vi "模拟时钟.vi"() -> ()   [LabVIEW 2016]
panel:
  out "时钟绘图":picture
  out "时间字符串":string
types:
  T1 = cluster{"Width":u16, "Style":enum32{"Solid", "Dash", "Dot", "DashDot", "DashDotDot"}}
  T2 = typedef "LVBoundsTypeDef.ctl" = cluster{"Width":u32, "Height":u32}
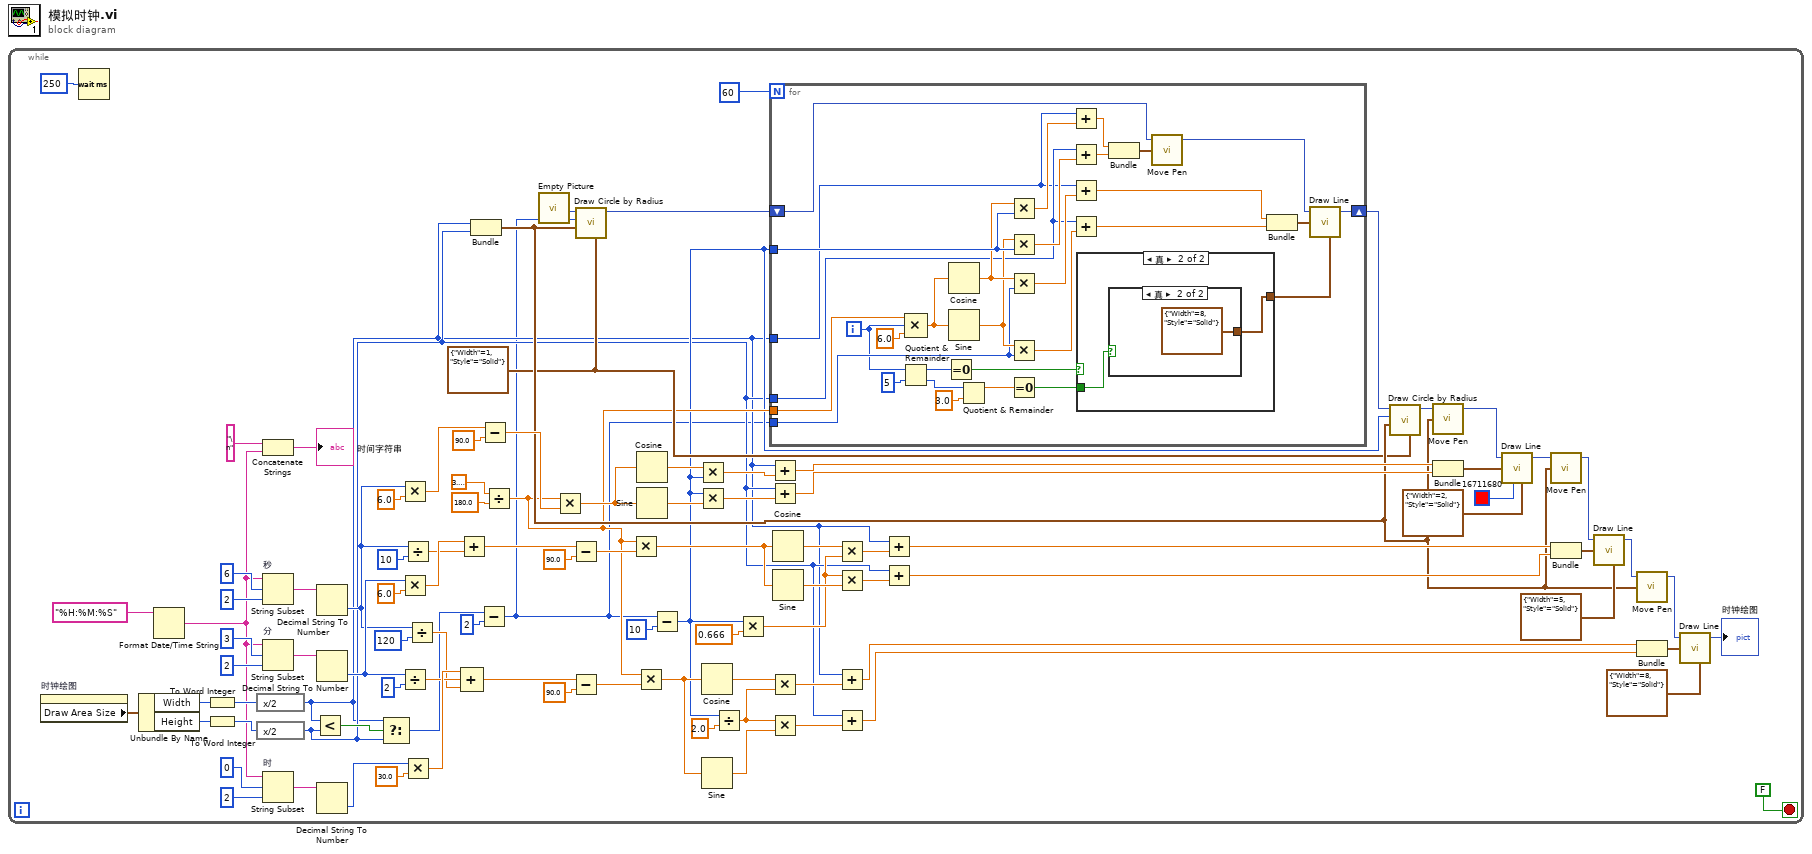
[diagram p0: block diagram]
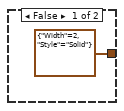
[diagram p2: hidden frame]
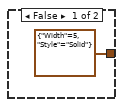
[diagram p3: hidden frame]
diagram:
  n1 = while {
    stop <- FALSE stop-if-true
    w14 = T1 {"Width"=1, "Style"=enum."Solid"} ("pen")
    n2 = property on="时钟绘图" class="Pict"() -> ("Draw Area Size"=w97:T2)  [unwired: 2 in, 2 out]
    n3 = Wait (ms)(milliseconds to wait=u32 250 ("等待时间（毫秒）")) -> ()  [unwired: 1 out]
    n4 = Unbundle By Name(w97) -> ("Width"=w93:u32, "Height"=w92:u32)
    n5 = Format Date/Time String(time format string (%c)="%H:%M:%S" ("时间格式字符串(%c)")) -> (date/time string=w3:string)  [unwired: 2 in]
    n6 = To Word Integer(number=w93) -> (16bit integer=w90:i16)
    n7 = To Word Integer(number=w92) -> (16bit integer=w89:i16)
    n8 = expression code="x/2"(w90) -> (w7:i16)
    n9 = expression code="x/2"(w89) -> (w8:i16)
    n10 = Concatenate Strings("\n" ("字符串"), w3) -> (→"时间字符串":string)
    n11 = String Subset "秒"(string=w3, offset (0)=6 ("偏移量(0)"), length (rest)=2 ("长度（剩余）")) -> (substring=w78:string)
    n12 = String Subset "分"(string=w3, offset (0)=3 ("偏移量(0)"), length (rest)=2 ("长度（剩余）")) -> (substring=w81:string)
    n13 = String Subset "时"(string=w3, offset (0)=0 ("偏移量(0)"), length (rest)=2 ("长度（剩余）")) -> (substring=w73:string)
    n14 = Less?(x=w7, y=w8) -> (x < y?=w94:bool)
    n15 = Decimal String To Number(string=w78) -> (number=w31:i32)  [unwired: 2 in, 1 out]
    n16 = Decimal String To Number(string=w81) -> (number=w35:i32)  [unwired: 2 in, 1 out]
    n17 = Decimal String To Number(string=w73) -> (number=w36:i32)  [unwired: 2 in, 1 out]
    n18 = Select(t=w7, s=w94, f=w8) -> (s? t:f=w13:i16)
    n19 = Multiply(x=w31, y=6.0) -> (x*y=w68:dbl)
    n20 = Multiply(x=w35, y=6.0) -> (x*y=w61:dbl)
    n21 = Divide(x=w35, y=2) -> (x/y=w33:dbl)
    n22 = Divide(x=w31, y=10) -> (x/y=w60:dbl)
    n23 = Multiply(x=w36, y=30.0) -> (x*y=w37:dbl)
    n24 = Divide(x=w31, y=120) -> (x/y=w32:dbl)
    n25 = Add(x=w61, y=w60) -> (x+y=w62:dbl)
    n26 = Compound Arithmetic op=ADD(w37, w33, w32) -> (w39:dbl)
    n27 = Bundle(w7, w8) -> (w15:cluster{i16, i16})  [unwired: 1 in]
    n28 = Subtract(x=w13, y=i16 2) -> (x-y=w6:i16)
    n29 = Subtract(x=w68, y=90.0) -> (x-y=w71:dbl)
    n30 = Divide(x=3.141592653589793, y=180.0) -> (x/y=w10:dbl)
    n31 = call "Empty Picture"() -> ("empty picture"=w16:picture)
    n32 = Multiply(x=w10, y=w71) -> (x*y=w82:dbl)
    n33 = Subtract(x=w62, y=90.0) -> (x-y=w65:dbl)
    n34 = Subtract(x=w39, y=90.0) -> (x-y=w42:dbl)
    n35 = call <vilib>:"Draw Circle by Radius.vi"("pen"=w14, "pixel center"=w15, "radius"=w6, "picture"=w16) -> ("new picture"=w5:picture)  [unwired: 7 in]
    n36 = Multiply(x=w10, y=w65) -> (x*y=w50:dbl)
    n37 = Multiply(x=w10, y=w42) -> (x*y=w49:dbl)
    n38 = Cosine(x=w82) -> (cos(x)=w86:dbl)
    n39 = Sine(x=w82) -> (sin(x)=w88:dbl)
    n40 = Subtract(x=w6, y=i16 10) -> (x-y=w9:i16)
    n41 = Multiply(x=w86, y=w9) -> (x*y=w85:dbl)
    n42 = Multiply(x=w9, y=w88) -> (x*y=w87:dbl)
    n43 = Cosine(x=w49) -> (cos(x)=w44:dbl)
    n44 = Sine(x=w49) -> (sin(x)=w46:dbl)
    n45 = Divide(x=w9, y=2.0) -> (x/y=w22:dbl)
    n46 = Multiply(x=w9, y=0.666) -> (x*y=w20:dbl)
    n47 = for {
      N: 60 -> [_]
      tunnel: w10 -> [w130]
      tunnel: w9 -> [w127]
      tunnel: w8 -> [w112]
      tunnel: w7 -> [w111]
      tunnel: w6 -> [w120]
      shift-right: [w109] -> w4
      shift-left: w5 -> [w110]
      i -> [w105]
      n48 = Quotient & Remainder(x=w105, y=5) -> (x-y*floor(x/y)=w107:i32, floor(x/y)=w102:i32)
      n49 = Compound Arithmetic op=MULTIPLY(w130, w105, 6.0 ("y")) -> (w128:dbl)
      n50 = Equal To 0?(x=w107) -> (x = 0?=w106:bool)
      n51 = Cosine(x=w128) -> (cos(x)=w122:dbl)
      n52 = Sine(x=w128) -> (sin(x)=w121:dbl)
      n53 = Quotient & Remainder(x=w102, y=3.0) -> (x-y*floor(x/y)=w101:dbl)  [unwired: 1 out]
      n54 = Multiply(x=w122, y=w127) -> (x*y=w123:dbl)
      n55 = Multiply(x=w121, y=w127) -> (x*y=w126:dbl)
      n56 = Multiply(x=w122, y=w120) -> (x*y=w124:dbl)
      n57 = Multiply(x=w121, y=w120) -> (x*y=w125:dbl)
      n58 = Equal To 0?(x=w101) -> (x = 0?=w100:bool)
      n59 = Add(x=w111, y=w123) -> (x+y=w118:dbl)
      n60 = Add(x=w112, y=w126) -> (x+y=w117:dbl)
      n61 = Add(x=w111, y=w124) -> (x+y=w115:dbl)
      n62 = Add(x=w112, y=w125) -> (x+y=w114:dbl)
      n63 = case shown="真" w106 {
        tunnel: [T1 {"Width"=2, "Style"=enum."Solid"} ("pen") w133] -> w108
        tunnel: w100 -> [_ w132]
        frame False {
        }
        frame True {
          n64 = case shown="真" w132 {
            tunnel: [T1 {"Width"=5, "Style"=enum."Solid"} ("pen") T1 {"Width"=8, "Style"=enum."Solid"} ("pen")] -> w133
            frame False {
            }
            frame True {
            }
          }
        }
      }
      n65 = Bundle(w118, w117) -> (w119:cluster{dbl, dbl})  [unwired: 1 in]
      n66 = call <vilib>:"Move Pen.vi"("new position"=w119, "picture"=w110) -> ("new picture"=w113:picture)  [unwired: 3 in]
      n67 = Bundle(w115, w114) -> (w116:cluster{dbl, dbl})  [unwired: 1 in]
      n68 = call <vilib>:"Draw Line.vi"("picture"=w113, "end point"=w116, "pen"=w108) -> ("new picture"=w109:picture)  [unwired: 6 in]
    }
    n69 = Add(x=w7, y=w85) -> (x+y=w84:dbl)
    n70 = Add(x=w8, y=w87) -> (x+y=w83:dbl)
    n71 = Multiply(x=w44, y=w22) -> (x*y=w43:dbl)
    n72 = Multiply(x=w22, y=w46) -> (x*y=w45:dbl)
    n73 = Cosine(x=w50) -> (cos(x)=w56:dbl)
    n74 = Sine(x=w50) -> (sin(x)=w54:dbl)
    n75 = Multiply(x=w56, y=w20) -> (x*y=w57:dbl)
    n76 = Multiply(x=w20, y=w54) -> (x*y=w55:dbl)
    n77 = Add(x=w7, y=w43) -> (x+y=w47:dbl)
    n78 = Add(x=w8, y=w45) -> (x+y=w48:dbl)
    n79 = Add(x=w7, y=w57) -> (x+y=w53:dbl)
    n80 = Add(x=w8, y=w55) -> (x+y=w52:dbl)
    n81 = call <vilib>:"Draw Circle by Radius.vi"("pen"=w14, "pixel center"=w15, "radius"=w9, "picture"=w4) -> ("new picture"=w19:picture)  [unwired: 7 in]
    n82 = call <vilib>:"Move Pen.vi"("new position"=w15, "picture"=w19) -> ("new picture"=w99:picture)  [unwired: 3 in]
    n83 = Bundle(w84, w83) -> (w91:cluster{dbl, dbl})  [unwired: 1 in]
    n84 = call <vilib>:"Draw Line.vi"("picture"=w99, "end point"=w91, "color(black)"=u32 16711680, "pen"=T1 {"Width"=2, "Style"=enum."Solid"}) -> ("new picture"=w28:picture)  [unwired: 5 in]
    n85 = call <vilib>:"Move Pen.vi"("new position"=w15, "picture"=w28) -> ("new picture"=w29:picture)  [unwired: 3 in]
    n86 = Bundle(w53, w52) -> (w51:cluster{dbl, dbl})  [unwired: 1 in]
    n87 = call <vilib>:"Draw Line.vi"("picture"=w29, "end point"=w51, "pen"=T1 {"Width"=5, "Style"=enum."Solid"}) -> ("new picture"=w26:picture)  [unwired: 6 in]
    n88 = call <vilib>:"Move Pen.vi"("new position"=w15, "picture"=w26) -> ("new picture"=w27:picture)  [unwired: 3 in]
    n89 = Bundle(w47, w48) -> (w40:cluster{dbl, dbl})  [unwired: 1 in]
    n90 = call <vilib>:"Draw Line.vi"("picture"=w27, "end point"=w40, "pen"=T1 {"Width"=8, "Style"=enum."Solid"}) -> ("new picture"=→"时钟绘图":picture)  [unwired: 6 in]
  }
